vi "Autonomous Independent.vi"   [LabVIEW 2020]
doc: "This VI is called when autonomous begins, and will automatically be terminated when autonomous ends. You can carry out timed or sensor driven robot movement independently without needing to return to the caller."
uses:
  <vilib>/Rock Robotics/Network Tables/NT Read String.vi
  <vilib>/Rock Robotics/WPI/Utilities/WPI_GetSetVariantRefNum.vi
  Robot Global Data.vi
  <vilib>/Rock Robotics/WPI/RobotDrive/WPI_RobotDriveArcadeDrive_Standard(NoSaturation).vi
  <vilib>/Rock Robotics/Network Tables/NT Write Numeric Array.vi
panel:
  # "Be sure to right-click and choose Data Operations>>Make Current Value default if you want to save the array values with the VI"
types:
  T1 = typedef "WPI_MotorControlDeviceRef.ctl" = cluster{"DeviceStatus":errorcluster, "Type":T2, "PWM":cluster{"PWM Channel":T3, "DeadBand":T4}, "CAN":cluster{"Device Number":u8, "SetOutput VI Ref":variant, "GetOutput VI Ref":variant, "Enable VI Ref":variant, "Disable VI Ref":variant, "Data":variant}, "Invert":bool, "DIO PWM":cluster{"PWM \"Enable\" Channel":T3, "DIOChannel":T5, "PWM Rate":dbl}}
  T2 = typedef "WPI_MotorControlType.ctl" = enum16{"PWM", "CAN", "DIO PWM"}
  T3 = typedef "FPGA_DIOPWMChannel.ctl" = enum8{"PWM 0", "PWM 1", "PWM 2", "PWM 3", "PWM 4", "PWM 5", "PWM 6", "PWM 7", "PWM 8", "PWM 9", "PWM MXP 0", "PWM MXP 1", "PWM MXP 2", "PWM MXP 3", "PWM MXP 4", "PWM MXP 5", "PWM MXP 6", "PWM MXP 7", "PWM MXP 8", "PWM MXP 9", "Invalid"}
  T4 = typedef "WPI_PWMDeadband.ctl" = cluster{"Name":string, "maxPositivePwm":i32, "minPositivePwm":i32, "centerPwm":i32, "maxNegativePwm":i32, "minNegativePwm":i32, "angularRange":u16}
  T5 = typedef "FPGA_DIOChannel.ctl" = enum8{"DIO 0", "DIO 1", "DIO 2", "DIO 3", "DIO 4", "DIO 5", "DIO 6", "DIO 7", "DIO 8", "DIO 9", "DIO MXP 0", "DIO MXP 1", "DIO MXP 2", "DIO MXP 3", "DIO MXP 4", "DIO MXP 5", "DIO MXP 6", "DIO MXP 7", "DIO MXP 8", "DIO MXP 9", "DIO MXP 10", "DIO MXP 11", "DIO MXP 12", "DIO MXP 13", "DIO MXP 14", "DIO MXP 15", "SPI Port CS1", "SPI Port CS2", "SPI Port CS3", "SPI Port MISO", "SPI Port MOSI", "Invalid"}
  T6 = typedef "WPI_RobotDriveDevRef.ctl" = cluster{"DevStatus":errorcluster, "Motors[]":T1[], "Square Inputs":bool, "Max Output":dbl}
  T7 = typedef "ADIS16470 Device Reference.ctl" = cluster{"DevStatus":errorcluster, "Hardware Config":T8, "Calibration Complete":refnum<notifier>, "Status Reference":refnum<data-value>, "Data Reference":refnum<data-value>, "Sychronous Process VI":T11, "Cmd FIFO":refnum<k33>, "Source":T12, "Data FIFO":refnum<k33>, "Calibration Time (ms)":u32, "Data Reference":refnum<data-value>}
  T8 = typedef "ADIS16470 Hardware Configuration.ctl" = cluster{"SPI Clock Rate (Hz)":dbl, "IMU SPI Mode (3)":T9, "IMU Reset Pin":T5, "IMU SPI Bus":T10, "IMU Data Ready Pin":T5, "Stall Config":cluster{"Pow2BytesPerRead":u8, "StallTicks":u16, "CsToSclkTicks":u8}}
  T9 = typedef "WPI_SPIMode.ctl" = enum16{"Mode 0 (Clk Idle Low,Sample on Leading)", "Mode 1 (Clk Idle Low,Sample on Trailing)", "Mode 2 (Clk Idle High,Sample on Leading)", "Mode 3 (Clk Idle High,Sample on Trailing)"}
  T10 = typedef "spi_bus.ctl" = enum16{"SPI On-Board, CS0", "SPI On-Board, CS1", "SPI On-Board, CS2", "SPI On-Board, CS3", "SPI MXP", "Invalid"}
  T11 = typedef "ADIS16470 Process.ctl" = refnum<vi>
  T12 = typedef "FPGA_CounterEncoderSourceConvertionLVSourceType.ctl" = cluster{"DevStatus":errorcluster, "AnalogTriggerMode?":bool, "DigitalMode":cluster{"DIO Channel":T13}, "AnalogTriggerMode":cluster{"AnalogTriggerIndex":T14, "OutputType":T15}}
  T13 = typedef "FPGA_DIODigitalSourceChannel.ctl" = enum8{"DIO 0", "DIO 1", "DIO 2", "DIO 3", "DIO 4", "DIO 5", "DIO 6", "DIO 7", "DIO 8", "DIO 9", "DIO MXP 0", "DIO MXP 1", "DIO MXP 2", "DIO MXP 3", "DIO MXP 4", "DIO MXP 5", "DIO MXP 6", "DIO MXP 7", "DIO MXP 8", "DIO MXP 9", "DIO MXP 10", "DIO MXP 11", "DIO MXP 12", "DIO MXP 13", "DIO MXP 14", "DIO MXP 15", "SPI Port CS1", "SPI Port CS2", "SPI Port CS3", "SPI Port MISO", "SPI Port MOSI", "Disabled"}
  T14 = typedef "FPGA_AnalogTriggerIndex.ctl" = enum8{"Trig 0", "Trig 1", "Trig 2", "Trig 3", "Trig 4", "Trig 5", "Trig 6", "Trig 7", "Invalid"}
  T15 = typedef "FPGA_AnalogTriggerOutType.ctl" = enum16{"InWindow", "TriggerState", "Rising", "Falling"}
  T16 = typedef "WPI_JoystickDevRef.ctl" = cluster{"Device":T17}
  T17 = typedef "WPI_JoystickDeviceEnum.ctl" = enum16{"USB 0", "USB 1", "USB 2", "USB 3", "USB 4", "USB 5"}
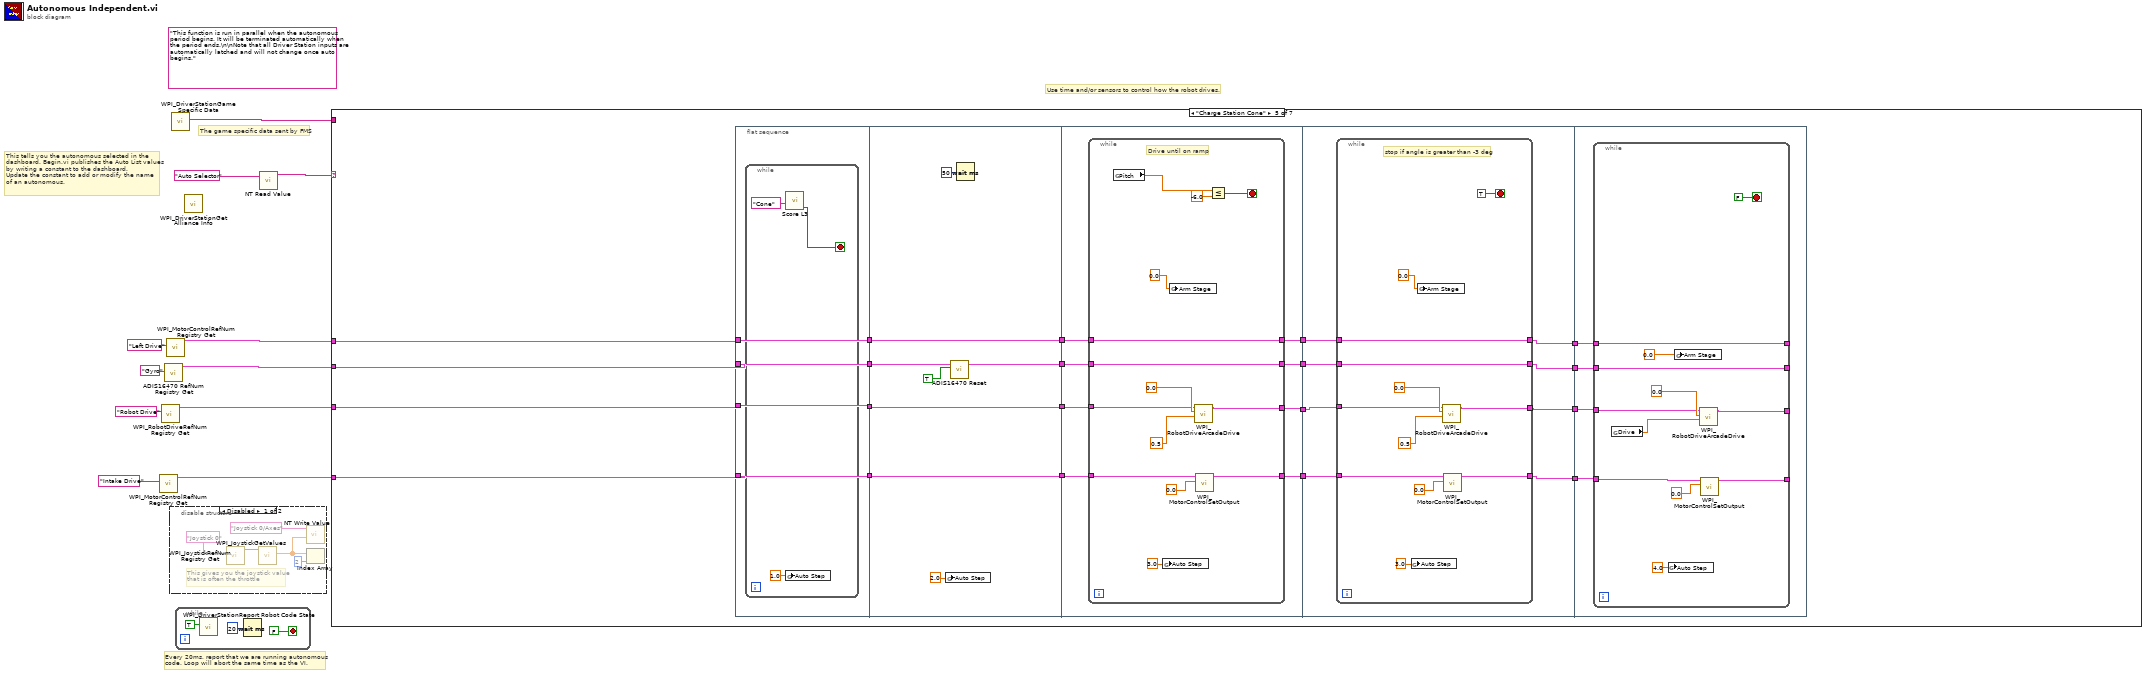
[diagram p0: block diagram]
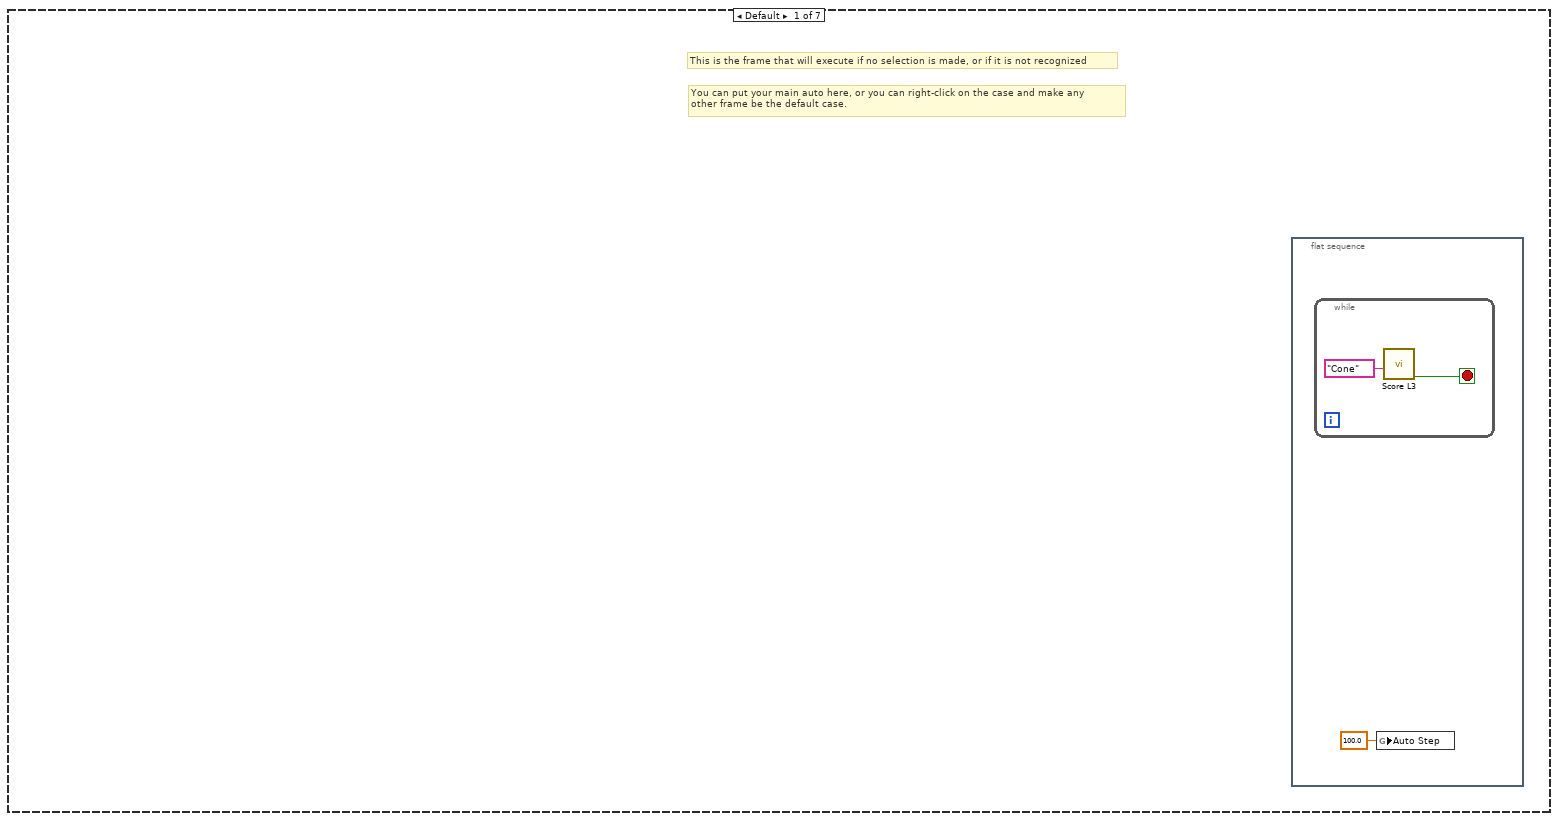
[diagram p3: hidden frame]
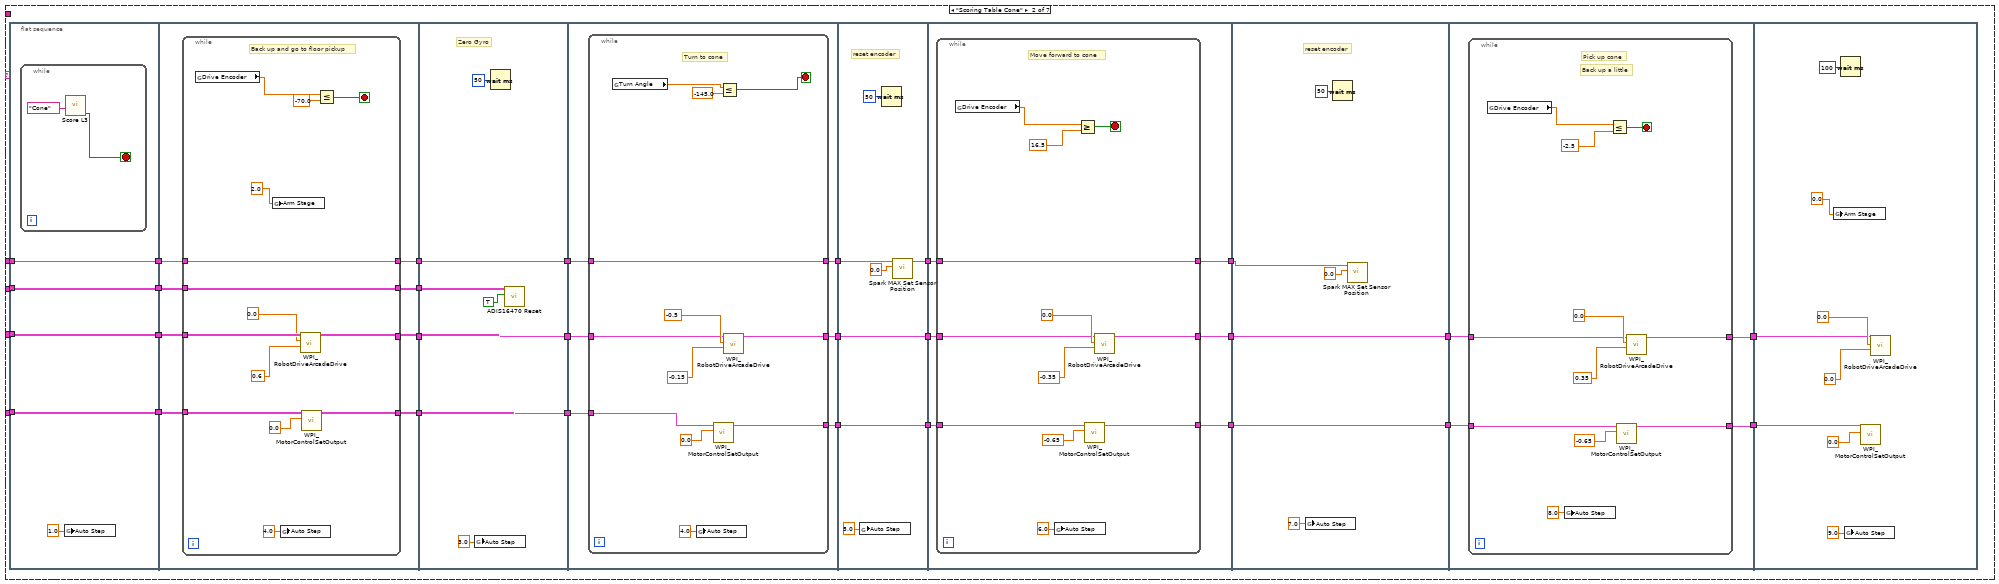
[diagram p4: hidden frame]
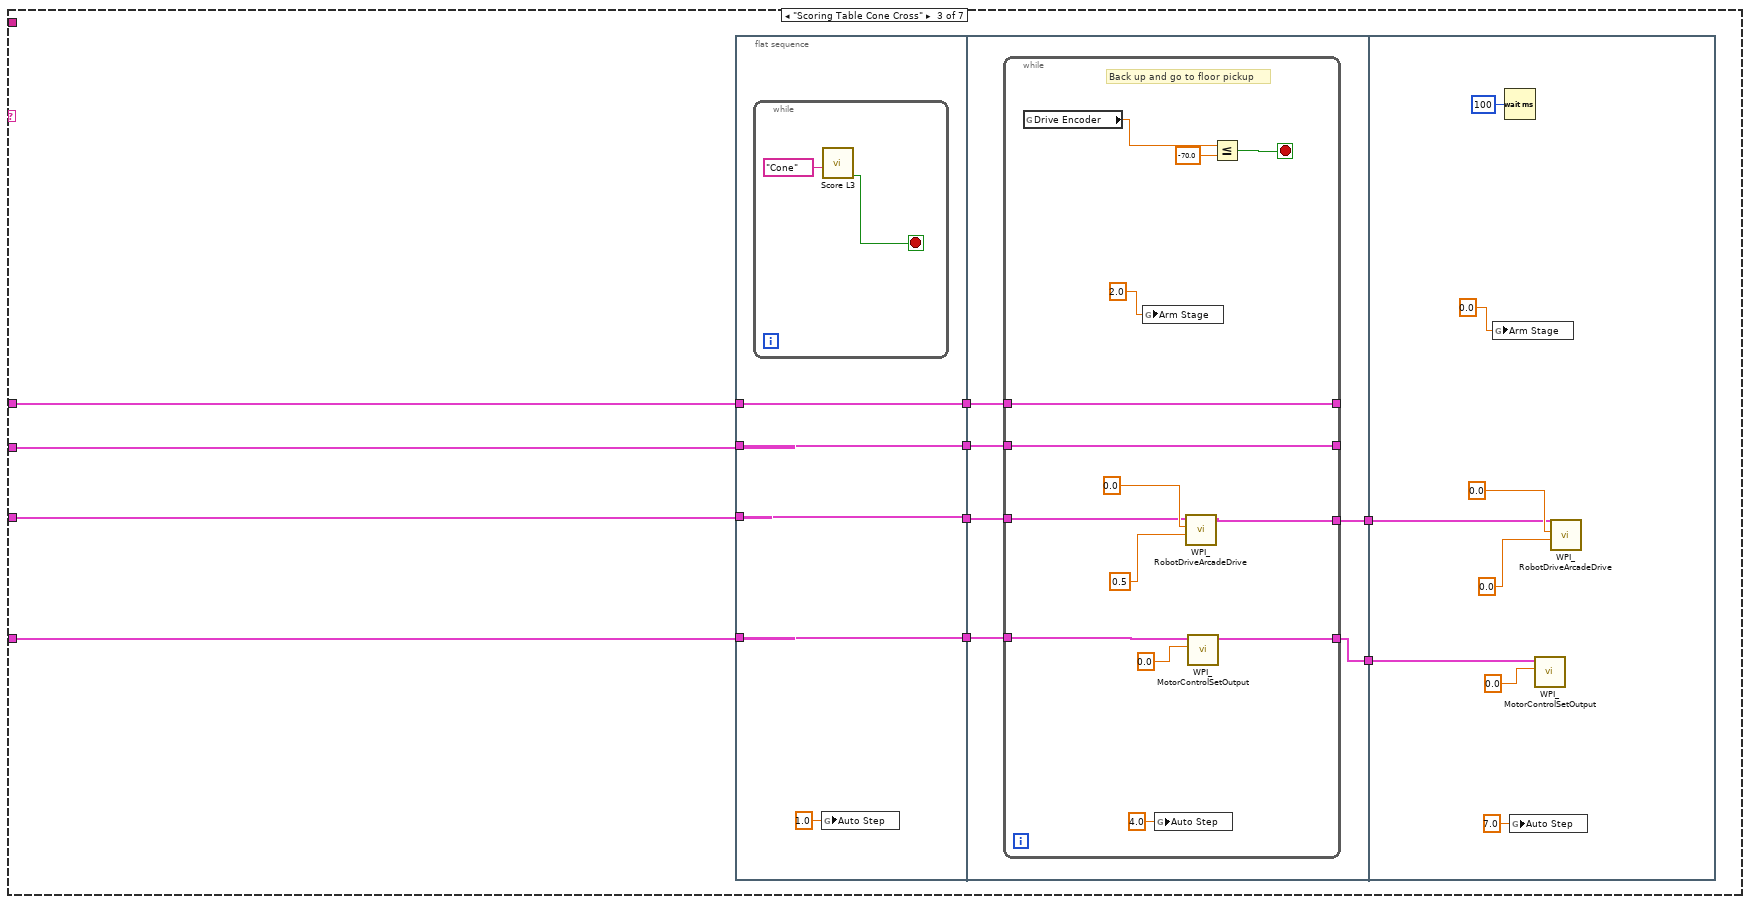
[diagram p5: hidden frame]
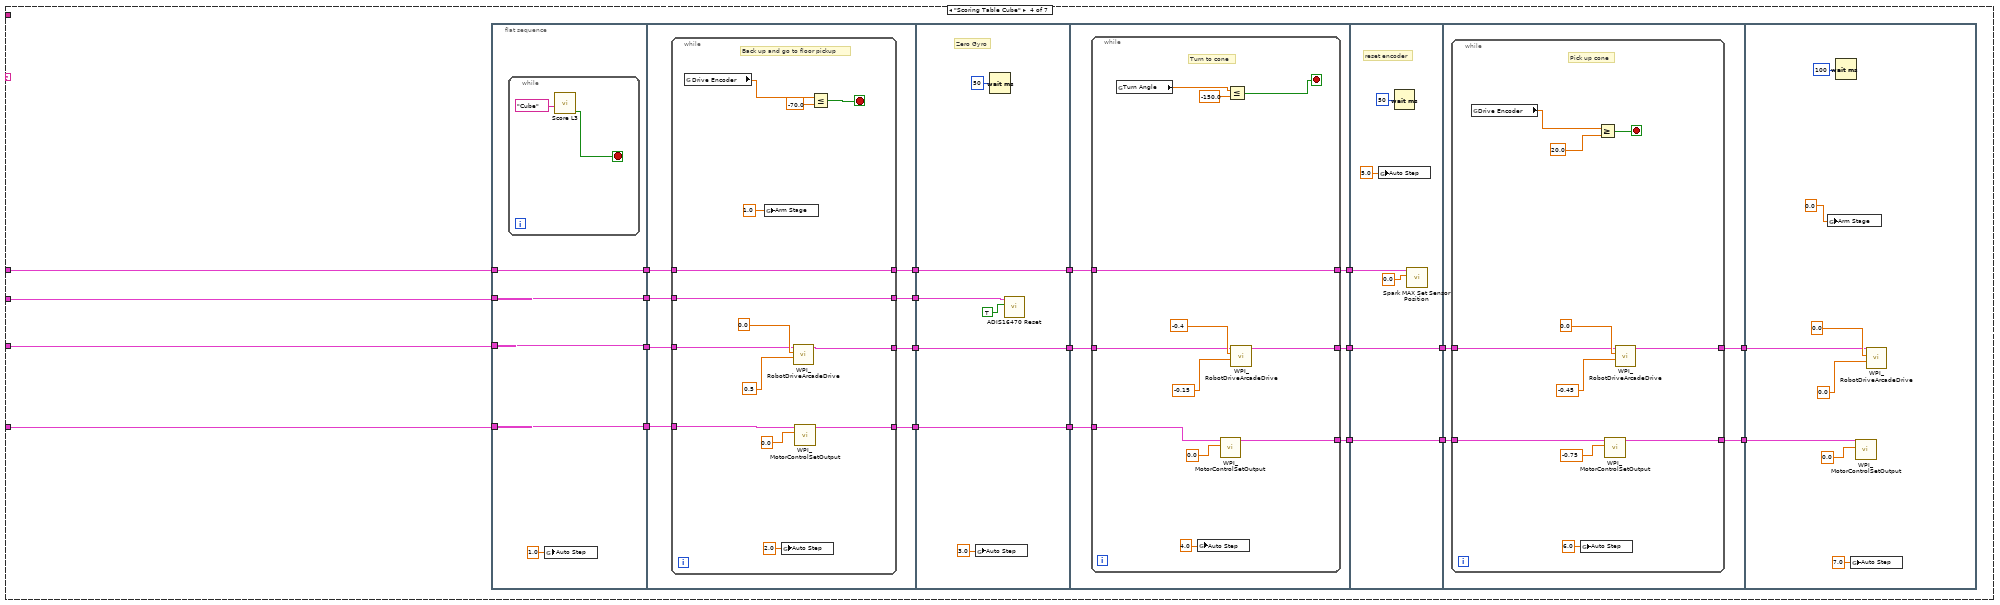
[diagram p6: hidden frame]
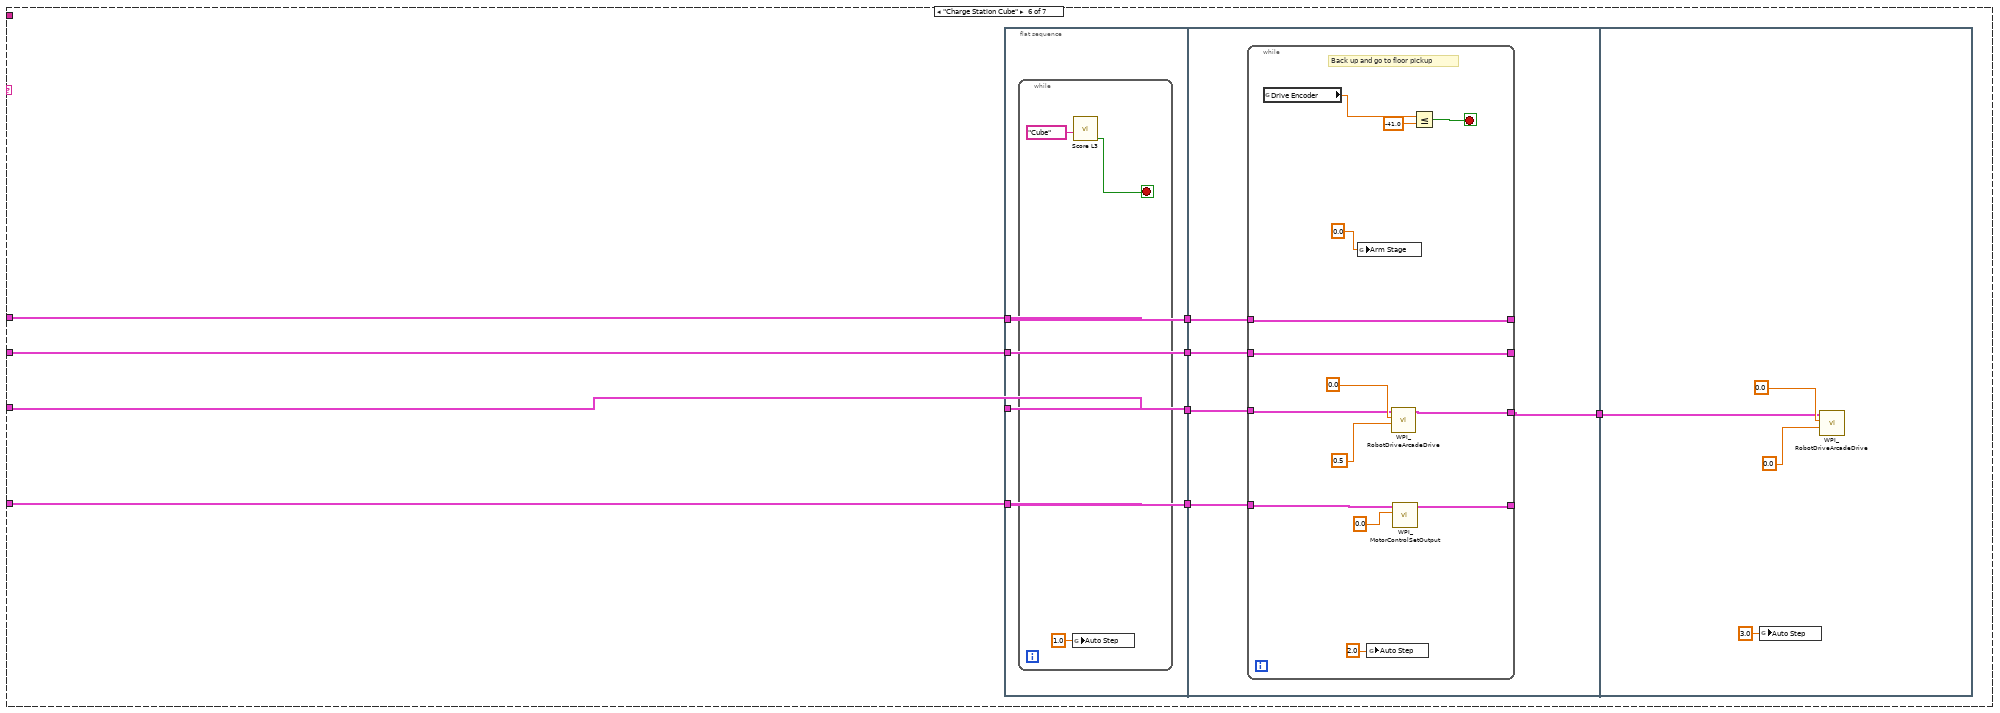
[diagram p7: hidden frame]
diagram:
  (unwired) "This function is run in parallel when the autonomous period begins. It will be terminated automatically when the period ends.\n\nNote that all Driver Station inputs are automatically latched and will not change once auto begins."
  # "The game specific data sent by FMS"
  # "This tells you the autonomous selected in the \ndashboard. Begin.vi publishes the Auto List values\nby writing a constant to the dashboard.\nUpdate the constant to add or modify the name\nof an autonomous."
  # "Every 20ms, report that we are running autonomous\ncode. Loop will abort the same time as the VI."
  # "Use time and/or sensors to control how the robot drives."
  n1 = call <vilib>:"WPI_MotorControlRefNum Registry Get.vi"("refnum name"="Intake Drive") -> ("MotorControlDevRef"=w1:T1)  [unwired: 9 in, 1 out]
  n2 = call <vilib>:"WPI_RobotDriveRefNum Registry Get.vi"("refnum name"="Robot Drive") -> ("RobotDriveDevRef"=w7:T6)  [unwired: 9 in, 1 out]
  n3 = call <vilib>:"ADIS16470 RefNum Registry Get.vi"("refnum name"="Gyro") -> ("ADIS16470DevRef out"=w3:T7)  [unwired: 9 in, 1 out]
  n4 = call <vilib>:"WPI_MotorControlRefNum Registry Get.vi"("refnum name"="Left Drive") -> ("MotorControlDevRef"=w4:T1)  [unwired: 9 in, 1 out]
  n5 = disable-structure shown="Disabled" {
    frame Disabled {
      # "This gives you the joystick value\nthat is often the throttle"
      n6 = call <vilib>:"WPI_JoystickRefNum Registry Get.vi"("refnum name"="Joystick 0") -> ("JoystickDevRef"=w15:T16)  [unwired: 1 in, 9 out]
      n7 = call <vilib>:"WPI_JoystickGetValues.vi"("JoystickDevRef"=w15) -> ("Axes"=w13:dbl[])  [unwired: 6 in, 4 out]
      n8 = call-poly <vilib>:"NT Write Value.vi"("value"=w13, "name"="Joystick 0/Axes" ("Name")) -> ()  [unwired: 9 in, 1 out]
      n9 = Index Array(array=w13, index=2) -> ()  [unwired: 1 out]
    }
    frame Enabled {
    }
  }
  n10 = call <vilib>:"WPI_DriverStationGame Specific Data.vi"() -> ("Game Specific Data"=w9:string)  [unwired: 11 in]
  n11 = while {
    stop <- FALSE stop-if-true
    n12 = call <vilib>:"WPI_DriverStationReport Robot Code State.vi"("Autonomous"=TRUE) -> ()  [unwired: 10 in, 1 out]
    n13 = Wait (ms)(milliseconds to wait=u32 20) -> ()  [unwired: 1 out]
  }
  n14 = call <vilib>:"WPI_DriverStationGet Alliance Info.vi"() -> ()  [unwired: 12 out]
  n15 = call-poly <vilib>:"NT Read Value.vi"("name"="Auto Selector" ("Name")) -> ("value"=w10:string)  [unwired: 8 in, 2 out]
  n16 = case shown="\"Charge Station Cone\"" w10 {
    tunnel: w9 -> [_ _ _ _ _ _ _]
    tunnel: w7 -> [_ w32 w162 w205 w326 w403 _]
    tunnel: w4 -> [_ w34 w164 w207 w328 w405 _]
    tunnel: w3 -> [_ w33 w163 w206 w327 w404 _]
    tunnel: w1 -> [_ w31 w161 w204 w325 w402 _]
    frame Default {
      # "You can put your main auto here, or you can right-click on the case and make any\nother frame be the default case."
      # "This is the frame that will execute if no selection is made, or if it is not recognized"
      n17 = flat-sequence {
        frame #0 {
          n18 = while {
            stop <- w22 stop-if-true
            n19 = call "Score L3.vi"("Combo Box"="Cone") -> ("Done"=w22:bool)  [unwired: 10 in]
          }
          n20 = global write "Robot Global Data.vi" "Auto Step"(100.0 ("Auto Step")) -> ()
        }
      }
    }
    frame "Scoring Table Cone" {
      n21 = flat-sequence {
        tunnel: [w53] -> w38
        tunnel: [w52] -> w37
        tunnel: [w54] -> w36
        tunnel: [w55] -> w35
        tunnel: w34 -> [w55]
        tunnel: w33 -> [w54]
        tunnel: w32 -> [w53]
        tunnel: w31 -> [w52]
        tunnel: w38 -> [w65]
        tunnel: w37 -> [w64]
        tunnel: [w63] -> w50
        tunnel: [w62] -> w48
        tunnel: [w61] -> w46
        tunnel: w36 -> [w60]
        tunnel: [w59] -> w43
        tunnel: w35 -> [w58]
        tunnel: w50 -> [w86]
        tunnel: [w86] -> w49
        tunnel: w48 -> [w85]
        tunnel: [w85] -> w47
        tunnel: w46 -> [w83]
        tunnel: [w81] -> w44
        tunnel: w43 -> [w81]
        tunnel: w49 -> [w92]
        tunnel: w47 -> [w91]
        tunnel: [w90] -> w45
        tunnel: w44 -> [w89]
        tunnel: [w88] -> w41
        tunnel: [w87] -> w39
        tunnel: w45 -> [w109]
        tunnel: [w108] -> w42
        tunnel: w41 -> [w108]
        tunnel: [w107] -> w40
        tunnel: w39 -> [w107]
        tunnel: [w105] -> w24
        tunnel: w42 -> [w117]
        tunnel: w40 -> [w116]
        tunnel: [w115] -> w28
        tunnel: [w114] -> w26
        tunnel: w24 -> [w113]
        tunnel: [w112] -> w23
        tunnel: w28 -> [w135]
        tunnel: [w135] -> w27
        tunnel: w26 -> [w134]
        tunnel: [w134] -> w25
        tunnel: w23 -> [w132]
        tunnel: w27 -> [w139]
        tunnel: [w137] -> w30
        tunnel: w25 -> [w138]
        tunnel: [w136] -> w29
        tunnel: w30 -> [w154]
        tunnel: w29 -> [w153]
        frame #0 {
          n22 = while {
            stop <- w57 stop-if-true
            n23 = call "Score L3.vi"("Combo Box"="Cone") -> ("Done"=w57:bool)  [unwired: 10 in]
          }
          n24 = global write "Robot Global Data.vi" "Auto Step"(1.0 ("Auto Step")) -> ()
        }
        frame #1 {
          n25 = while {
            tunnel: w65 -> [w76]
            tunnel: w64 -> [w75]
            tunnel: [w70] -> w63
            tunnel: [w69] -> w62
            tunnel: [w68] -> w61
            tunnel: w60 -> [w68]
            tunnel: [w67] -> w59
            tunnel: w58 -> [w67]
            stop <- w72 stop-if-true
            # "Back up and go to floor pickup"
            n26 = global read "Robot Global Data.vi" "Drive Encoder"() -> (w74:dbl)
            n27 = global write "Robot Global Data.vi" "Arm Stage"(2.0 ("Arm Stage")) -> ()
            n28 = global write "Robot Global Data.vi" "Auto Step"(4.0 ("Auto Step")) -> ()
            n29 = call-poly <vilib>:"WPI_RobotDriveArcadeDrive.vi"("Y axis value"=0.6, "X axis value"=0.0, "RobotDriveDevRef"=w76) -> ("RobotDriveDevRef"=w69:T6)  [unwired: 6 in, 2 out]
            n30 = call <vilib>:"WPI_MotorControlSetOutput.vi"("Output"=0.0, "MotorControlDevRef"=w75) -> ("MotorControlDevRef"=w70:T1)  [unwired: 7 in, 2 out]
            n31 = Less Or Equal?(x=w74, y=-70.0) -> (x <= y?=w72:bool)
          }
        }
        frame #2 {
          # "Zero Gyro"
          n32 = global write "Robot Global Data.vi" "Auto Step"(3.0 ("Auto Step")) -> ()
          n33 = Wait (ms)(milliseconds to wait=u32 50) -> ()  [unwired: 1 out]
          n34 = call <vilib>:"ADIS16470 Reset.vi"("Reset? (T)"=TRUE, "ADIS16470DevRef"=w83) -> ()  [unwired: 8 in, 2 out]
        }
        frame #3 {
          n35 = while {
            tunnel: w92 -> [w99]
            tunnel: w91 -> [w98]
            tunnel: [w96] -> w90
            tunnel: w89 -> [w96]
            tunnel: [w95] -> w88
            tunnel: [w94] -> w87
            stop <- w103 stop-if-true
            # "Turn to cone"
            n36 = global read "Robot Global Data.vi" "Turn Angle"() -> (w97:dbl)
            n37 = global write "Robot Global Data.vi" "Auto Step"(4.0 ("Auto Step")) -> ()
            n38 = call <vilib>:"WPI_MotorControlSetOutput.vi"("Output"=0.0, "MotorControlDevRef"=w99) -> ("MotorControlDevRef"=w94:T1)  [unwired: 7 in, 2 out]
            n39 = Less Or Equal?(x=w97, y=-145.0) -> (x <= y?=w103:bool)
            n40 = call-poly <vilib>:"WPI_RobotDriveArcadeDrive.vi"("Y axis value"=-0.15, "X axis value"=-0.5, "RobotDriveDevRef"=w98) -> ("RobotDriveDevRef"=w95:T6)  [unwired: 6 in, 2 out]
          }
        }
        frame #4 {
          # "reset encoder"
          n41 = global write "Robot Global Data.vi" "Auto Step"(5.0 ("Auto Step")) -> ()
          n42 = Wait (ms)(milliseconds to wait=u32 50) -> ()  [unwired: 1 out]
          n43 = call <vilib>:"Spark MAX Set Sensor Position.vi"("Position"=0.0, "MotorControlDeviceRef"=w109) -> ("MotorControlDeviceRef"=w105:T1)  [unwired: 8 in, 1 out]
        }
        frame #5 {
          n44 = while {
            tunnel: w117 -> [w126]
            tunnel: w116 -> [w125]
            tunnel: [w121] -> w115
            tunnel: [w120] -> w114
            tunnel: w113 -> [w118]
            tunnel: [w118] -> w112
            stop <- w122 stop-if-true
            # "Move forward to cone"
            n45 = global read "Robot Global Data.vi" "Drive Encoder"() -> (w124:dbl)
            n46 = global write "Robot Global Data.vi" "Auto Step"(6.0 ("Auto Step")) -> ()
            n47 = Greater Or Equal?(x=w124, y=16.5) -> (x >= y?=w122:bool)
            n48 = call <vilib>:"WPI_MotorControlSetOutput.vi"("Output"=-0.65, "MotorControlDevRef"=w125) -> ("MotorControlDevRef"=w120:T1)  [unwired: 7 in, 2 out]
            n49 = call-poly <vilib>:"WPI_RobotDriveArcadeDrive.vi"("Y axis value"=-0.35, "X axis value"=0.0, "RobotDriveDevRef"=w126) -> ("RobotDriveDevRef"=w121:T6)  [unwired: 6 in, 2 out]
          }
        }
        frame #6 {
          # "reset encoder"
          n50 = global write "Robot Global Data.vi" "Auto Step"(7.0 ("Auto Step")) -> ()
          n51 = Wait (ms)(milliseconds to wait=u32 50) -> ()  [unwired: 1 out]
          n52 = call <vilib>:"Spark MAX Set Sensor Position.vi"("Position"=0.0, "MotorControlDeviceRef"=w132) -> ()  [unwired: 8 in, 2 out]
        }
        frame #7 {
          n53 = while {
            tunnel: w139 -> [w147]
            tunnel: w138 -> [w146]
            tunnel: [w142] -> w137
            tunnel: [w141] -> w136
            stop <- w143 stop-if-true
            # "Back up a little"
            # "Pick up cone"
            n54 = global read "Robot Global Data.vi" "Drive Encoder"() -> (w145:dbl)
            n55 = global write "Robot Global Data.vi" "Auto Step"(8.0 ("Auto Step")) -> ()
            n56 = Less Or Equal?(x=w145, y=-2.5) -> (x <= y?=w143:bool)
            n57 = call <vilib>:"WPI_MotorControlSetOutput.vi"("Output"=-0.65, "MotorControlDevRef"=w146) -> ("MotorControlDevRef"=w141:T1)  [unwired: 7 in, 2 out]
            n58 = call-poly <vilib>:"WPI_RobotDriveArcadeDrive.vi"("Y axis value"=0.35, "X axis value"=0.0, "RobotDriveDevRef"=w147) -> ("RobotDriveDevRef"=w142:T6)  [unwired: 6 in, 2 out]
          }
        }
        frame #8 {
          n59 = global write "Robot Global Data.vi" "Arm Stage"(0.0 ("Arm Stage")) -> ()
          n60 = Wait (ms)(milliseconds to wait=u32 100) -> ()  [unwired: 1 out]
          n61 = global write "Robot Global Data.vi" "Auto Step"(9.0 ("Auto Step")) -> ()
          n62 = call <vilib>:"WPI_MotorControlSetOutput.vi"("Output"=0.0, "MotorControlDevRef"=w153) -> ()  [unwired: 7 in, 3 out]
          n63 = call-poly <vilib>:"WPI_RobotDriveArcadeDrive.vi"("Y axis value"=0.0, "X axis value"=0.0, "RobotDriveDevRef"=w154) -> ()  [unwired: 6 in, 3 out]
        }
      }
    }
    frame "Scoring Table Cone Cross" {
      n64 = flat-sequence {
        tunnel: [w171] -> w168
        tunnel: [w170] -> w167
        tunnel: [w172] -> w166
        tunnel: [w173] -> w165
        tunnel: w164 -> [w173]
        tunnel: w163 -> [w172]
        tunnel: w162 -> [w171]
        tunnel: w161 -> [w170]
        tunnel: w168 -> [w181]
        tunnel: w167 -> [w180]
        tunnel: w166 -> [w179]
        tunnel: w165 -> [w178]
        tunnel: [w177] -> w160
        tunnel: [w176] -> w159
        tunnel: w160 -> [w197]
        tunnel: w159 -> [w196]
        frame #0 {
          n65 = while {
            stop <- w175 stop-if-true
            n66 = call "Score L3.vi"("Combo Box"="Cone") -> ("Done"=w175:bool)  [unwired: 10 in]
          }
          n67 = global write "Robot Global Data.vi" "Auto Step"(1.0 ("Auto Step")) -> ()
        }
        frame #1 {
          n68 = while {
            tunnel: w181 -> [w192]
            tunnel: w180 -> [w191]
            tunnel: [w186] -> w176
            tunnel: [w185] -> w177
            tunnel: [w184] -> _
            tunnel: w179 -> [w184]
            tunnel: [w183] -> _
            tunnel: w178 -> [w183]
            stop <- w188 stop-if-true
            # "Back up and go to floor pickup"
            n69 = global read "Robot Global Data.vi" "Drive Encoder"() -> (w190:dbl)
            n70 = global write "Robot Global Data.vi" "Arm Stage"(2.0 ("Arm Stage")) -> ()
            n71 = global write "Robot Global Data.vi" "Auto Step"(4.0 ("Auto Step")) -> ()
            n72 = call-poly <vilib>:"WPI_RobotDriveArcadeDrive.vi"("Y axis value"=0.5, "X axis value"=0.0, "RobotDriveDevRef"=w192) -> ("RobotDriveDevRef"=w185:T6)  [unwired: 6 in, 2 out]
            n73 = call <vilib>:"WPI_MotorControlSetOutput.vi"("Output"=0.0, "MotorControlDevRef"=w191) -> ("MotorControlDevRef"=w186:T1)  [unwired: 7 in, 2 out]
            n74 = Less Or Equal?(x=w190, y=-70.0) -> (x <= y?=w188:bool)
          }
        }
        frame #2 {
          n75 = global write "Robot Global Data.vi" "Arm Stage"(0.0 ("Arm Stage")) -> ()
          n76 = Wait (ms)(milliseconds to wait=u32 100) -> ()  [unwired: 1 out]
          n77 = global write "Robot Global Data.vi" "Auto Step"(7.0 ("Auto Step")) -> ()
          n78 = call <vilib>:"WPI_MotorControlSetOutput.vi"("Output"=0.0, "MotorControlDevRef"=w196) -> ()  [unwired: 7 in, 3 out]
          n79 = call-poly <vilib>:"WPI_RobotDriveArcadeDrive.vi"("Y axis value"=0.0, "X axis value"=0.0, "RobotDriveDevRef"=w197) -> ()  [unwired: 6 in, 3 out]
        }
      }
    }
    frame "Scoring Table Cube" {
      n80 = flat-sequence {
        tunnel: [w228] -> w211
        tunnel: [w227] -> w210
        tunnel: [w229] -> w209
        tunnel: [w230] -> w208
        tunnel: w207 -> [w230]
        tunnel: w206 -> [w229]
        tunnel: w205 -> [w228]
        tunnel: w204 -> [w227]
        tunnel: w211 -> [w240]
        tunnel: w210 -> [w239]
        tunnel: [w238] -> w225
        tunnel: [w237] -> w223
        tunnel: [w236] -> w221
        tunnel: w209 -> [w235]
        tunnel: [w234] -> w218
        tunnel: w208 -> [w233]
        tunnel: w225 -> [w261]
        tunnel: [w261] -> w224
        tunnel: w223 -> [w260]
        tunnel: [w260] -> w222
        tunnel: w221 -> [w258]
        tunnel: [w256] -> w219
        tunnel: w218 -> [w256]
        tunnel: w224 -> [w267]
        tunnel: w222 -> [w266]
        tunnel: [w265] -> w220
        tunnel: w219 -> [w264]
        tunnel: [w263] -> w216
        tunnel: [w262] -> w214
        tunnel: w220 -> [w283]
        tunnel: [w282] -> w217
        tunnel: w216 -> [w282]
        tunnel: [w281] -> w215
        tunnel: w214 -> [w281]
        tunnel: w217 -> [w289]
        tunnel: w215 -> [w288]
        tunnel: [w287] -> w213
        tunnel: [w286] -> w212
        tunnel: w213 -> [w304]
        tunnel: w212 -> [w303]
        frame #0 {
          n81 = while {
            stop <- w232 stop-if-true
            n82 = call "Score L3.vi"("Combo Box"="Cube") -> ("Done"=w232:bool)  [unwired: 10 in]
          }
          n83 = global write "Robot Global Data.vi" "Auto Step"(1.0 ("Auto Step")) -> ()
        }
        frame #1 {
          n84 = while {
            tunnel: w240 -> [w251]
            tunnel: w239 -> [w250]
            tunnel: [w245] -> w238
            tunnel: [w244] -> w237
            tunnel: [w243] -> w236
            tunnel: w235 -> [w243]
            tunnel: [w242] -> w234
            tunnel: w233 -> [w242]
            stop <- w247 stop-if-true
            # "Back up and go to floor pickup"
            n85 = global read "Robot Global Data.vi" "Drive Encoder"() -> (w249:dbl)
            n86 = global write "Robot Global Data.vi" "Arm Stage"(1.0 ("Arm Stage")) -> ()
            n87 = global write "Robot Global Data.vi" "Auto Step"(2.0 ("Auto Step")) -> ()
            n88 = call-poly <vilib>:"WPI_RobotDriveArcadeDrive.vi"("Y axis value"=0.5, "X axis value"=0.0, "RobotDriveDevRef"=w251) -> ("RobotDriveDevRef"=w244:T6)  [unwired: 6 in, 2 out]
            n89 = call <vilib>:"WPI_MotorControlSetOutput.vi"("Output"=0.0, "MotorControlDevRef"=w250) -> ("MotorControlDevRef"=w245:T1)  [unwired: 7 in, 2 out]
            n90 = Less Or Equal?(x=w249, y=-70.0) -> (x <= y?=w247:bool)
          }
        }
        frame #2 {
          # "Zero Gyro"
          n91 = global write "Robot Global Data.vi" "Auto Step"(3.0 ("Auto Step")) -> ()
          n92 = Wait (ms)(milliseconds to wait=u32 50) -> ()  [unwired: 1 out]
          n93 = call <vilib>:"ADIS16470 Reset.vi"("Reset? (T)"=TRUE, "ADIS16470DevRef"=w258) -> ()  [unwired: 8 in, 2 out]
        }
        frame #3 {
          n94 = while {
            tunnel: w267 -> [w274]
            tunnel: w266 -> [w273]
            tunnel: [w271] -> w265
            tunnel: w264 -> [w271]
            tunnel: [w270] -> w263
            tunnel: [w269] -> w262
            stop <- w278 stop-if-true
            # "Turn to cone"
            n95 = global read "Robot Global Data.vi" "Turn Angle"() -> (w272:dbl)
            n96 = global write "Robot Global Data.vi" "Auto Step"(4.0 ("Auto Step")) -> ()
            n97 = call <vilib>:"WPI_MotorControlSetOutput.vi"("Output"=0.0, "MotorControlDevRef"=w274) -> ("MotorControlDevRef"=w269:T1)  [unwired: 7 in, 2 out]
            n98 = Less Or Equal?(x=w272, y=-150.0) -> (x <= y?=w278:bool)
            n99 = call-poly <vilib>:"WPI_RobotDriveArcadeDrive.vi"("Y axis value"=-0.15, "X axis value"=-0.4, "RobotDriveDevRef"=w273) -> ("RobotDriveDevRef"=w270:T6)  [unwired: 6 in, 2 out]
          }
        }
        frame #4 {
          # "reset encoder"
          n100 = global write "Robot Global Data.vi" "Auto Step"(5.0 ("Auto Step")) -> ()
          n101 = Wait (ms)(milliseconds to wait=u32 50) -> ()  [unwired: 1 out]
          n102 = call <vilib>:"Spark MAX Set Sensor Position.vi"("Position"=0.0, "MotorControlDeviceRef"=w283) -> ()  [unwired: 8 in, 2 out]
        }
        frame #5 {
          n103 = while {
            tunnel: w289 -> [w297]
            tunnel: w288 -> [w296]
            tunnel: [w292] -> w287
            tunnel: [w291] -> w286
            stop <- w293 stop-if-true
            # "Pick up cone"
            n104 = global read "Robot Global Data.vi" "Drive Encoder"() -> (w295:dbl)
            n105 = global write "Robot Global Data.vi" "Auto Step"(6.0 ("Auto Step")) -> ()
            n106 = Greater Or Equal?(x=w295, y=20.0) -> (x >= y?=w293:bool)
            n107 = call <vilib>:"WPI_MotorControlSetOutput.vi"("Output"=-0.75, "MotorControlDevRef"=w296) -> ("MotorControlDevRef"=w291:T1)  [unwired: 7 in, 2 out]
            n108 = call-poly <vilib>:"WPI_RobotDriveArcadeDrive.vi"("Y axis value"=-0.45, "X axis value"=0.0, "RobotDriveDevRef"=w297) -> ("RobotDriveDevRef"=w292:T6)  [unwired: 6 in, 2 out]
          }
        }
        frame #6 {
          n109 = global write "Robot Global Data.vi" "Arm Stage"(0.0 ("Arm Stage")) -> ()
          n110 = Wait (ms)(milliseconds to wait=u32 100) -> ()  [unwired: 1 out]
          n111 = global write "Robot Global Data.vi" "Auto Step"(7.0 ("Auto Step")) -> ()
          n112 = call <vilib>:"WPI_MotorControlSetOutput.vi"("Output"=0.0, "MotorControlDevRef"=w303) -> ()  [unwired: 7 in, 3 out]
          n113 = call-poly <vilib>:"WPI_RobotDriveArcadeDrive.vi"("Y axis value"=0.0, "X axis value"=0.0, "RobotDriveDevRef"=w304) -> ()  [unwired: 6 in, 3 out]
        }
      }
    }
    frame "Charge Station Cone" {
      n114 = flat-sequence {
        tunnel: [w330] -> w323
        tunnel: [w329] -> w321
        tunnel: [w331] -> w319
        tunnel: [w332] -> w318
        tunnel: w328 -> [w332]
        tunnel: w327 -> [w331]
        tunnel: w326 -> [w330]
        tunnel: w325 -> [w329]
        tunnel: w323 -> [w343]
        tunnel: [w343] -> w322
        tunnel: w321 -> [w342]
        tunnel: [w342] -> w320
        tunnel: w319 -> [w337]
        tunnel: w318 -> [w341]
        tunnel: [w341] -> w317
        tunnel: [w338] -> w316
        tunnel: w322 -> [w349]
        tunnel: w320 -> [w348]
        tunnel: w317 -> [w351]
        tunnel: [w347] -> w324
        tunnel: w316 -> [w350]
        tunnel: [w346] -> w315
        tunnel: [w345] -> w314
        tunnel: [w344] -> w313
        tunnel: w324 -> [w371]
        tunnel: w315 -> [w373]
        tunnel: w314 -> [w372]
        tunnel: w313 -> [w370]
        tunnel: [w369] -> w312
        tunnel: [w368] -> w311
        tunnel: [w367] -> w310
        tunnel: [w366] -> w309
        tunnel: w312 -> [w388]
        tunnel: w311 -> [w389]
        tunnel: w310 -> [w387]
        tunnel: w309 -> [w386]
        frame #0 {
          n115 = while {
            stop <- w335 stop-if-true
            n116 = global write "Robot Global Data.vi" "Auto Step"(1.0 ("Auto Step")) -> ()
            n117 = call "Score L3.vi"("Combo Box"="Cone") -> ("Done"=w335:bool)  [unwired: 10 in]
          }
        }
        frame #1 {
          n118 = global write "Robot Global Data.vi" "Auto Step"(2.0 ("Auto Step")) -> ()
          n119 = call <vilib>:"ADIS16470 Reset.vi"("Reset? (T)"=TRUE, "ADIS16470DevRef"=w337) -> ("ADIS16470DevRef"=w338:T7)  [unwired: 8 in, 1 out]
          n120 = Wait (ms)(milliseconds to wait=u32 50) -> ()  [unwired: 1 out]
        }
        frame #2 {
          n121 = while {
            tunnel: w349 -> [w362]
            tunnel: w348 -> [w361]
            tunnel: [w356] -> w344
            tunnel: [w355] -> w347
            tunnel: [w354] -> w345
            tunnel: w350 -> [w354]
            tunnel: [w353] -> w346
            tunnel: w351 -> [w353]
            stop <- w358 stop-if-true
            # "Drive until on ramp"
            n122 = global read "Robot Global Data.vi" "Pitch"() -> (w360:dbl)
            n123 = global write "Robot Global Data.vi" "Auto Step"(3.0 ("Auto Step")) -> ()
            n124 = global write "Robot Global Data.vi" "Arm Stage"(0.0 ("Arm Stage")) -> ()
            n125 = call-poly <vilib>:"WPI_RobotDriveArcadeDrive.vi"("Y axis value"=0.5, "X axis value"=0.0, "RobotDriveDevRef"=w362) -> ("RobotDriveDevRef"=w355:T6)  [unwired: 6 in, 2 out]
            n126 = call <vilib>:"WPI_MotorControlSetOutput.vi"("Output"=0.0, "MotorControlDevRef"=w361) -> ("MotorControlDevRef"=w356:T1)  [unwired: 7 in, 2 out]
            n127 = Less Or Equal?(x=w360, y=-6.0) -> (x <= y?=w358:bool)
          }
        }
        frame #3 {
          n128 = while {
            tunnel: w371 -> [w382]
            tunnel: w370 -> [w381]
            tunnel: [w379] -> w368
            tunnel: [w378] -> w369
            tunnel: [w377] -> w367
            tunnel: w372 -> [w377]
            tunnel: [w376] -> w366
            tunnel: w373 -> [w376]
            stop <- TRUE stop-if-true
            # "stop if angle is greater than -3 deg"
            n129 = global write "Robot Global Data.vi" "Auto Step"(3.0 ("Auto Step")) -> ()
            n130 = global write "Robot Global Data.vi" "Arm Stage"(0.0 ("Arm Stage")) -> ()
            n131 = call-poly <vilib>:"WPI_RobotDriveArcadeDrive.vi"("Y axis value"=0.5, "X axis value"=0.0, "RobotDriveDevRef"=w382) -> ("RobotDriveDevRef"=w378:T6)  [unwired: 6 in, 2 out]
            n132 = call <vilib>:"WPI_MotorControlSetOutput.vi"("Output"=0.0, "MotorControlDevRef"=w381) -> ("MotorControlDevRef"=w379:T1)  [unwired: 7 in, 2 out]
          }
        }
        frame #4 {
          n133 = while {
            tunnel: w388 -> [w399]
            tunnel: w389 -> [w398]
            tunnel: [w396] -> _
            tunnel: [w395] -> _
            tunnel: [w394] -> _
            tunnel: w387 -> [w394]
            tunnel: [w393] -> _
            tunnel: w386 -> [w393]
            stop <- FALSE stop-if-true
            n134 = global read "Robot Global Data.vi" "Drive"() -> (w390:dbl)
            n135 = global write "Robot Global Data.vi" "Auto Step"(4.0 ("Auto Step")) -> ()
            n136 = global write "Robot Global Data.vi" "Arm Stage"(0.0 ("Arm Stage")) -> ()
            n137 = call-poly <vilib>:"WPI_RobotDriveArcadeDrive.vi"("Y axis value"=w390, "X axis value"=0.0, "RobotDriveDevRef"=w399) -> ("RobotDriveDevRef"=w395:T6)  [unwired: 6 in, 2 out]
            n138 = call <vilib>:"WPI_MotorControlSetOutput.vi"("Output"=0.0, "MotorControlDevRef"=w398) -> ("MotorControlDevRef"=w396:T1)  [unwired: 7 in, 2 out]
          }
        }
      }
    }
    frame "Charge Station Cube" {
      n139 = flat-sequence {
        tunnel: [w412] -> w410
        tunnel: [w411] -> w409
        tunnel: [w413] -> w408
        tunnel: [w414] -> w407
        tunnel: w405 -> [w414]
        tunnel: w404 -> [w413]
        tunnel: w403 -> [w412]
        tunnel: w402 -> [w411]
        tunnel: w410 -> [w420]
        tunnel: w409 -> [w419]
        tunnel: w408 -> [w421]
        tunnel: w407 -> [w422]
        tunnel: [w418] -> w406
        tunnel: w406 -> [w438]
        frame #0 {
          n140 = while {
            stop <- w417 stop-if-true
            n141 = global write "Robot Global Data.vi" "Auto Step"(1.0 ("Auto Step")) -> ()
            n142 = call "Score L3.vi"("Combo Box"="Cube") -> ("Done"=w417:bool)  [unwired: 10 in]
          }
        }
        frame #1 {
          n143 = while {
            tunnel: w420 -> [w433]
            tunnel: w419 -> [w432]
            tunnel: [w427] -> _
            tunnel: [w426] -> w418
            tunnel: [w425] -> _
            tunnel: w421 -> [w425]
            tunnel: [w424] -> _
            tunnel: w422 -> [w424]
            stop <- w429 stop-if-true
            # "Back up and go to floor pickup"
            n144 = global read "Robot Global Data.vi" "Drive Encoder"() -> (w431:dbl)
            n145 = global write "Robot Global Data.vi" "Arm Stage"(0.0 ("Arm Stage")) -> ()
            n146 = global write "Robot Global Data.vi" "Auto Step"(2.0 ("Auto Step")) -> ()
            n147 = call-poly <vilib>:"WPI_RobotDriveArcadeDrive.vi"("Y axis value"=0.5, "X axis value"=0.0, "RobotDriveDevRef"=w433) -> ("RobotDriveDevRef"=w426:T6)  [unwired: 6 in, 2 out]
            n148 = call <vilib>:"WPI_MotorControlSetOutput.vi"("Output"=0.0, "MotorControlDevRef"=w432) -> ("MotorControlDevRef"=w427:T1)  [unwired: 7 in, 2 out]
            n149 = Less Or Equal?(x=w431, y=-41.0) -> (x <= y?=w429:bool)
          }
        }
        frame #2 {
          n150 = global write "Robot Global Data.vi" "Auto Step"(3.0 ("Auto Step")) -> ()
          n151 = call-poly <vilib>:"WPI_RobotDriveArcadeDrive.vi"("Y axis value"=0.0, "X axis value"=0.0, "RobotDriveDevRef"=w438) -> ()  [unwired: 6 in, 3 out]
        }
      }
    }
    frame "Loading Station" {
      n152 = flat-sequence {
        frame #0 {
        }
        frame #1 {
        }
        frame #2 {
        }
        frame #3 {
        }
      }
    }
  }
